vi "USB Relay Control 256.vi"(8 "error in (no error)":errorcluster, 9 "Send to relay board":i32) -> (0 "error out":errorcluster)   [LabVIEW 2019]
uses:
  D2XX_Functions/D2XX_Functions.lvlib
panel:
  out "FT_Status 2":u32(ring) items=["FT_OK", "FT_INVALID_HANDLE", "FT_DEVICE_NOT_FOUND", "FT_DEVICE_NOT_OPENED", "FT_IO_ERROR", "FT_INSUFFICIENT_RESOURCES", "FT_INVALID_PARAMETER", "FT_INVALID_BAUD_RATE", "FT_DEVICE_NOT_OPENED_FOR_ERASE", "FT_DEVICE_NOT_OPENED_FOR_WRITE", "FT_FAILED_TO_WRITE_DEVICE", "FT_EEPROM_READ_FAILED", "FT_EEPROM_WRITE_FAILED", "FT_EEPROM_ERASE_FAILED", "FT_EEPROM_NOT_PRESENT", "FT_EEPROM_NOT_PROGRAMMED", "FT_INVALID_ARGS", "FT_NOT_SUPPORTED", "FT_OTHER_ERROR"]
  out "Device Description":string
  out "FT_Status":u32(ring) items=["FT_OK", "FT_INVALID_HANDLE", "FT_DEVICE_NOT_FOUND", "FT_DEVICE_NOT_OPENED", "FT_IO_ERROR", "FT_INSUFFICIENT_RESOURCES", "FT_INVALID_PARAMETER", "FT_INVALID_BAUD_RATE", "FT_DEVICE_NOT_OPENED_FOR_ERASE", "FT_DEVICE_NOT_OPENED_FOR_WRITE", "FT_FAILED_TO_WRITE_DEVICE", "FT_EEPROM_READ_FAILED", "FT_EEPROM_WRITE_FAILED", "FT_EEPROM_ERASE_FAILED", "FT_EEPROM_NOT_PRESENT", "FT_EEPROM_NOT_PROGRAMMED", "FT_INVALID_ARGS", "FT_NOT_SUPPORTED", "FT_OTHER_ERROR"]
  out "Port Index":string
  # "Number between 0 and 255,\nwhose binary representation\nis what relays will be on or off"
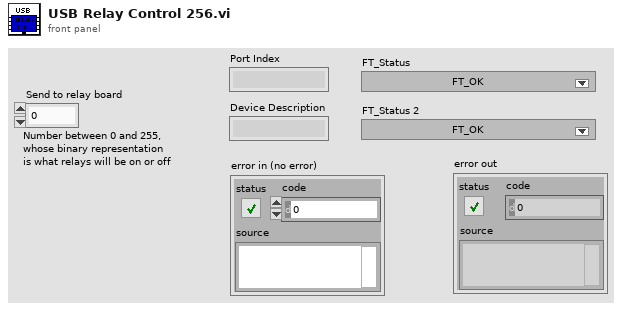
[diagram p1: front panel]
types:
  T1 = cluster{"Signature 1":u32, "Signature 2":u32, "Version":u32, "Vendor ID":u16, "Product ID":u16, "Manufacturer":string, "Manufacturer ID":string, "Description":string, "Serial Number":string, "Max Power (mA)":u16, "PnP":u16, "Self Powered":u16, "Remote Wake-Up":u16, "Rev4":u8, "Iso In":u8, "Iso Out":u8, "Pull Down Enable":u8, "Serial Number Enable":u8, "USB Version Enable":u8, "USB Version":u16, "Rev5":u8, "Iso In A":u8, "Iso In B":u8, "Iso Out A":u8, "Iso Out B":u8, "Pull Down Enable 5":u8, "Serial Number Enable 5":u8, "USB Version Enable 5":u8, "USB Version 5":u16, "A Is High Current":u8, "B Is High Current":u8, "A Is 245 FIFO":u8, "A Is CPU FIFO":u8, "A Is Fast Serial":u8, "A Is VCP":u8, "B Is 245 FIFO":u8, "B Is CPU FIFO":u8, "B Is Fast Serial":u8, "B Is VCP":u8, "Use Ext Osc":u8, "High Drive IOs":u8, "Endpoint Size":u8, "Pull Down Enable R":u8, "Serial Number Enable R":u8, "Invert TXD":u8, "Invert RXD":u8, "Invert RTS":u8, "Invert CTS":u8, "Invert DTR":u8, "Invert DSR":u8, "Invert DCD":u8, "Invert RI":u8, "CBus0":u8, "CBus1":u8, "CBus2":u8, "CBus3":u8, "CBus4":u8, "R Is VCP":u8, "Pull Down Enable 7":u8, "Serial Number Enable 7":u8, "AL Slow Slew":u8, "AL Schmitt Input":u8, "AL Drive Current":u8, "AH Slow Slew":u8, "AH Schmitt Input":u8, "AH Drive Current":u8, "BL Slow Slew":u8, "BL Schmitt Input":u8, "BL Drive Current":u8, "BH Slow Slew":u8, "BH Schmitt Input":u8, "BH Drive Current":u8, "A Is 245 FIFO 7":u8, "A Is CPU FIFO 7":u8, "A Is Fast Serial 7":u8, "A Is VCP 7":u8, "B Is 245 FIFO 7":u8, "B Is CPU FIFO 7":u8, "B Is Fast Serial 7":u8, "B Is VCP 7":u8, "PowerSaveEnable":u8, "Pull Down Enable 8":u8, "Serial Number Enable 8":u8, "A Slow Slew":u8, "A Schmitt Input":u8, "A Drive Current":u8, "B Slow Slew":u8, "B Schmitt Input":u8, "B Drive Current":u8, "C Slow Slew":u8, "C Schmitt Input":u8, "C Drive Current":u8, "D Slow Slew":u8, "D Schmitt Input":u8, "D Drive Current":u8, "A RI Is TXDEN":u8, "B RI Is TXDEN":u8, "C RI Is TXDEN":u8, "D RI Is TXDEN":u8, "A Is VCP 8":u8, "B Is VCP 8":u8, "C Is VCP 8":u8, "D Is VCP 8":u8}
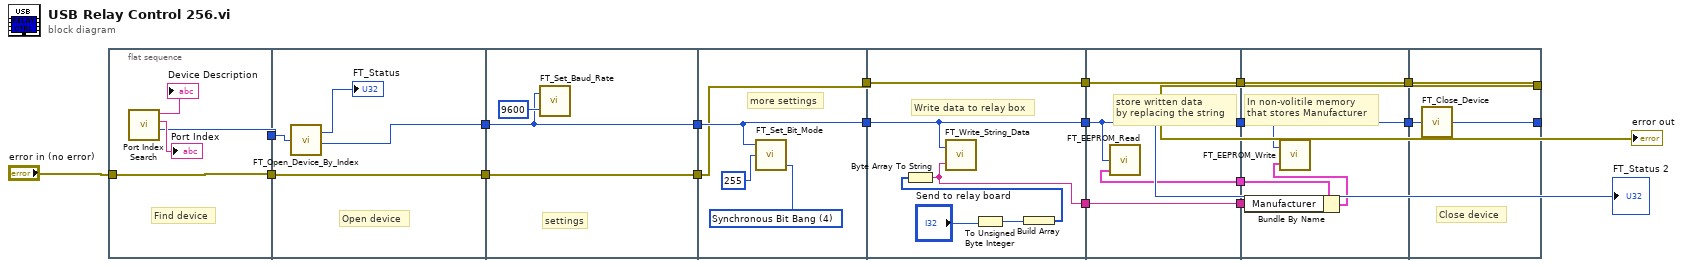
[diagram p0: block diagram]
diagram:
  n1 = flat-sequence {
    tunnel: [w21] -> w20
    tunnel: "error in (no error)" -> [w22]
    tunnel: [w22] -> w15
    tunnel: w20 -> [w27]
    tunnel: [w25] -> w18
    tunnel: [w26] -> w16
    tunnel: w15 -> [w26]
    tunnel: [w29] -> w11
    tunnel: w18 -> [w29]
    tunnel: [w30] -> w10
    tunnel: w16 -> [w30]
    tunnel: w11 -> [w33]
    tunnel: [w33] -> w13
    tunnel: w10 -> [w32]
    tunnel: [w32] -> w12
    tunnel: w13 -> [w40]
    tunnel: [w40] -> w9
    tunnel: [w41] -> w8
    tunnel: w12 -> [w41]
    tunnel: [w36] -> w1
    tunnel: w9 -> [w44]
    tunnel: [w44] -> w7
    tunnel: w8 -> [w45]
    tunnel: [w45] -> w5
    tunnel: [w43] -> w3
    tunnel: [w42] -> w2
    tunnel: w1 -> [w42]
    tunnel: w7 -> [w49]
    tunnel: [w49] -> w6
    tunnel: w5 -> [w50]
    tunnel: [w50] -> w4
    tunnel: w3 -> [w48]
    tunnel: w2 -> [w46]
    tunnel: w6 -> [w52]
    tunnel: [w53] -> w19
    tunnel: [w51] -> w14
    tunnel: w4 -> [w51]
    frame #0 {
      # "Find device"
      n2 = call "Port Index Search.vi"() -> ("Decimal Port Index"=w21:i32, "Port Index"=→"Port Index":string, "Device Description"=→"Device Description":string)  [unwired: 8 in, 1 out]
    }
    frame #1 {
      # "Open device"
      n3 = call "FT_Open_Device_By_Index.vi"("Device Index"=w27) -> ("FT_Status"=→"FT_Status":u32, "Handle"=w25:u32)
    }
    frame #2 {
      # "settings"
      n4 = call "FT_Set_Baud_Rate.vi"("Baud Rate"=u32 9600, "Handle"=w29) -> ()  [unwired: 1 out]
    }
    frame #3 {
      w35 = u8 4 items=["Reset Bit Mode"=0, "Asynchronous Bit Bang"=1, "MPSSE"=2, "Synchronous Bit Bang"=4, "MCU Host Bus Emulation"=8, "Fast Opto-Isolated Serial"=16, "CBUS Bit Bang"=32, "Single Channel 245 Synchronous FIFO"=64] ("Bit Mode")
      # "more settings"
      n5 = call "FT_Set_Bit_Mode.vi"("Bit Mode"=w35, "Bit Mode Mask"=u8 255, "Handle"=w33) -> ()  [unwired: 1 out]
    }
    frame #4 {
      # "Write data to relay box"
      n6 = To Unsigned Byte Integer(number="Send to relay board") -> (unsigned 8bit integer=w38:u8)
      n7 = Build Array(w38) -> (w37:u8[])
      n8 = Byte Array To String(unsigned byte array=w37) -> (string=w36:string)
      n9 = call "FT_Write_String_Data.vi"("Buffer"=w36, "Handle"=w40) -> ()  [unwired: 2 out]
    }
    frame #5 {
      # "store written data\nby replacing the string"
      n10 = call "FT_EEPROM_Read.vi"("Handle"=w44) -> ("output cluster"=w43:T1)  [unwired: 2 out]
    }
    frame #6 {
      # "In non-volitile memory\nthat stores Manufacturer"
      n11 = Bundle By Name(cluster=w48, "Manufacturer"=w46) -> (w47:T1)
      n12 = call "FT_EEPROM_Write.vi"("FT232-FT245R EEPROM Contents"=w47, "Handle"=w49) -> ()  [unwired: 1 out]
    }
    frame #7 {
      # "Close device"
      n13 = call "FT_Close_Device.vi"("Handle"=w52) -> ("FT_Status"=w53:u32)
    }
  }
  "FT_Status 2" <- w19
  "error out" <- w14
